vi "get Damage.vi"(11 "Weapon in":refnum<class "Weapon.lvclass">) -> (3 "Damage":i32)   [LabVIEW 2021, in "Weapon.lvclass"]
uses:
  Weapon.lvclass
  Weapon.lvclass/Weapon.ctl
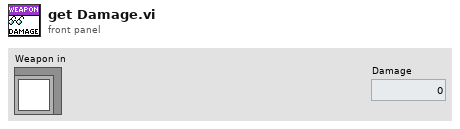
[diagram p1: front panel]
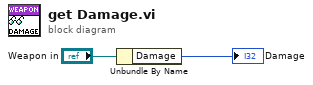
[diagram p0: block diagram]
diagram:
  n1 = Unbundle By Name("Weapon in") -> ("Damage"=→"Damage":i32)
